vi "Get Depth Image.vi"() -> ()   [LabVIEW 2011, in "LVH-Interface-for-Kinect.lvlib"]
uses:
  <vilib>/LabVIEW Hacker/LVH-Interface-for-Kinect/LVH-Interface-for-Kinect.lvlib
panel:
  out "Image":T1(plugin-control)
  out "error out":errorcluster
  in  "error in (no error)":errorcluster
  in  "Image Type":T2 items=["Grayscale (U8)", "Grayscale (I16)", "Grayscale (SGL)", "Complex (CSG)", "RGB (U32)", "HSL (U32)", "RGB (U64)", "Grayscale (U16)"]
  in  "Image Name":string="untitled"
  in  "Border Size":i32=3
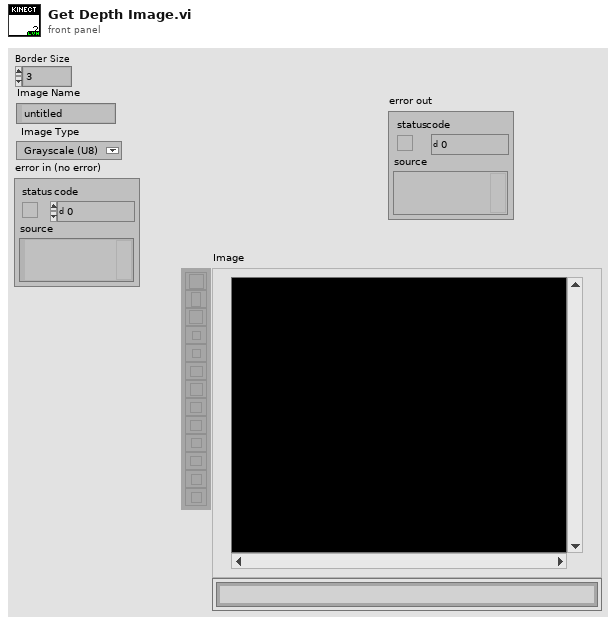
[diagram p1: front panel]
types:
  T1 = typedef "IMAQ Image.ctl" = refnum<image>
  T2 = typedef "Image Type" = u32
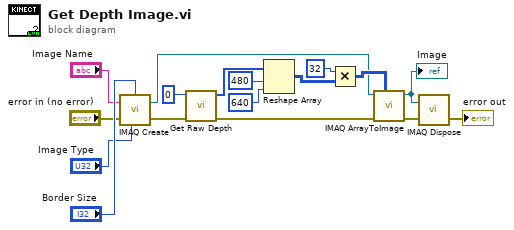
[diagram p0: block diagram]
diagram:
  n1 = call "IMAQ Create"("Border Size"="Border Size", "Image Name"="Image Name", "Image Type"="Image Type", "error in (no error)"="error in (no error)") -> ("New Image"=w7:T1, "error out"=w3:errorcluster)  [unwired: 1 in]
  n2 = call <vilib>:"Get Raw Depth.vi"("error in (no error)"=w3, "index"=0) -> ("error out"=w2:errorcluster, "Destination"=w8:u16[])  [unwired: 8 in]
  n3 = Reshape Array(w8, 480 ("dimension size"), 640 ("dimension size")) -> (w10:u16[][])
  n4 = Multiply(x=32, y=w10) -> (x*y=w9:i32[][])
  n5 = call "IMAQ ArrayToImage"("Image Pixels (U16)"=w9, "error in (no error)"=w2, "Image"=w7) -> ("error out"=w4:errorcluster, "Image Out"=w6:T1)  [unwired: 7 in]
  "Image" <- w6
  n6 = call "IMAQ Dispose"("Image"=w6, "error in (no error)"=w4) -> ("error out"=→"error out":errorcluster)  [unwired: 4 in]
